vi "Multiclamp Holding Potential Ramp.vi"(5 "Speed [mV/s]":dbl, 7 "Target [mV]":dbl, 8 "error in (no error)":errorcluster, 9 "pnError":i32, 11 "hMCCmsg":i32) -> (0 "error out":errorcluster, 1 "pnError out":i32, 3 "hMCCmsg OUT":i32)   [LabVIEW 2012, in "MultiClamp 700B Controls.lvlib"]
uses:
  MultiClamp 700B Controls.lvlib
  AxMultiClampMsg/AxMultiClampMsg.lvlib
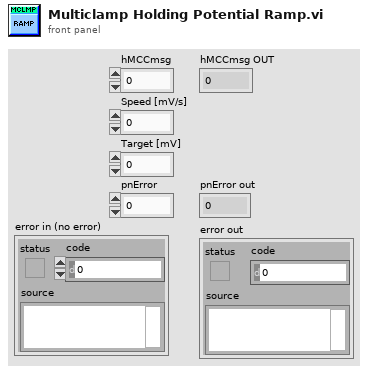
[diagram p1: front panel]
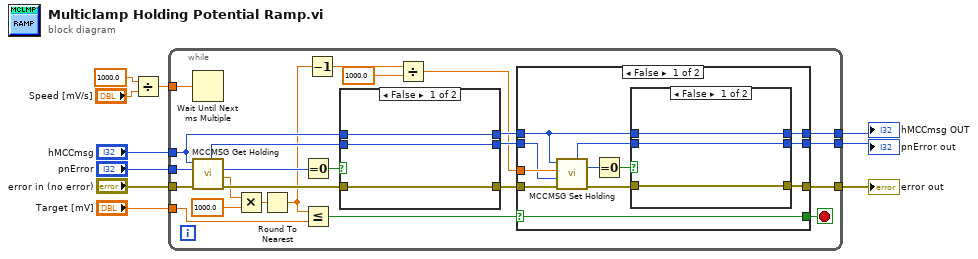
[diagram p0: block diagram]
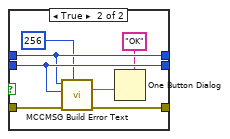
[diagram p2: hidden frame]
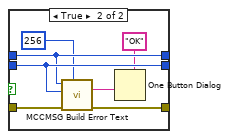
[diagram p3: hidden frame]
diagram:
  n1 = Divide(x=1000.0 ("y"), y="Speed [mV/s]") -> (x/y=w5:dbl)
  n2 = while {
    tunnel: w5 -> [w34]
    tunnel: "Target [mV]" -> [w15]
    tunnel: "hMCCmsg" -> [w29]
    tunnel: "pnError" -> [w28]
    tunnel: "error in (no error)" -> [w27]
    tunnel: [w21] -> w8
    tunnel: [w20] -> w7
    tunnel: [w19] -> w6
    stop <- w22 stop-if-true
    n3 = Wait Until Next ms Multiple(millisecond multiple=w34) -> ()  [unwired: 1 out]
    n4 = call "MCCMSG Get Holding.vi"("error in (no error)"=w27, "pnError"=w28, "hMCCmsg"=w29) -> ("error out"=w31:errorcluster, "pnError out"=w30:i32, "pdHolding out"=w16:dbl, "function return"=w32:i32)  [unwired: 5 in]
    n5 = Multiply(x=w16, y=1000.0) -> (x*y=w18:dbl)
    n6 = Round To Nearest(number=w18) -> (nearest integer value=w17:dbl)
    n7 = Equal To 0?(x=w32) -> (x = 0?=w33:bool)
    n8 = Less Or Equal?(x=w17, y=w15) -> (x <= y?=w25:bool)
    n9 = Decrement(x=w17) -> (x-1=w13:dbl)
    n10 = case shown="False" w33 {
      tunnel: w30 -> [w37 w43]
      tunnel: w31 -> [w35 w44]
      tunnel: w29 -> [w36 w42]
      tunnel: [w37 w43] -> w23
      tunnel: [w36 w42] -> w24
      tunnel: [w35 w38] -> w26
      frame False {
      }
      frame True {
        n11 = call "MCCMSG Build Error Text.vi"("uMaxLen"=u32 256, "error in (no error)"=w44, "nErrorNum"=w43, "hMCCmsg"=w42) -> ("error out"=w38:errorcluster, "sTxtBuf out"=w41:string)  [unwired: 5 in, 1 out]
        n12 = One Button Dialog(message=w41, button name ("OK")="OK") -> ()  [unwired: 1 out]
      }
    }
    n13 = Divide(x=w13, y=1000.0) -> (x/y=w11:dbl)
    n14 = case shown="False" w25 {
      selector: w25 -> [w45 w67]
      tunnel: w26 -> [w52 w68]
      tunnel: w11 -> [w51 _]
      tunnel: w24 -> [w50 w70]
      tunnel: w23 -> [w49 w69]
      tunnel: [w48 w70] -> w21
      tunnel: [w47 w69] -> w20
      tunnel: [w46 w68] -> w19
      tunnel: [w45 w67] -> w22
      frame False {
        n15 = call "MCCMSG Set Holding.vi"("error in (no error)"=w52, "pnError"=w49, "dHolding"=w51, "hMCCmsg"=w50) -> ("error out"=w55:errorcluster, "pnError out"=w53:i32, "function return"=w54:i32)  [unwired: 5 in]
        n16 = Equal To 0?(x=w54) -> (x = 0?=w56:bool)
        n17 = case shown="False" w56 {
          tunnel: w53 -> [w59 w65]
          tunnel: w55 -> [w57 w66]
          tunnel: w50 -> [w58 w64]
          tunnel: [w59 w65] -> w47
          tunnel: [w58 w64] -> w48
          tunnel: [w57 w60] -> w46
          frame False {
          }
          frame True {
            n18 = call "MCCMSG Build Error Text.vi"("uMaxLen"=u32 256, "error in (no error)"=w66, "nErrorNum"=w65, "hMCCmsg"=w64) -> ("error out"=w60:errorcluster, "sTxtBuf out"=w63:string)  [unwired: 5 in, 1 out]
            n19 = One Button Dialog(message=w63, button name ("OK")="OK") -> ()  [unwired: 1 out]
          }
        }
      }
      frame True {
      }
    }
  }
  "hMCCmsg OUT" <- w8
  "pnError out" <- w7
  "error out" <- w6
